vi "FirstOrderFilter.vi"(9 "fps":dbl, 10 "fc":dbl, 11 "Numeric in":dbl) -> (3 "Numeric out":dbl)   [LabVIEW 2017]
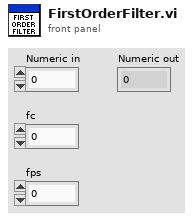
[diagram p1: front panel]
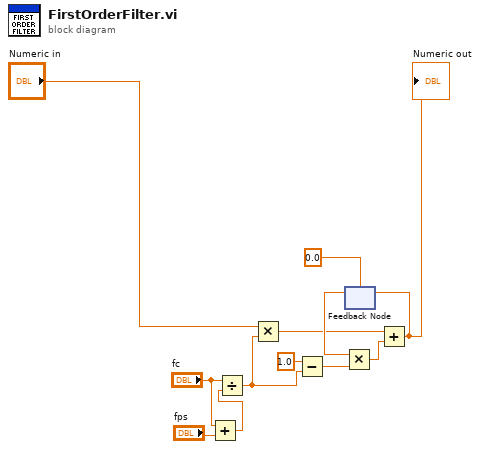
[diagram p0: block diagram]
diagram:
  n1 = Add(x="fc", y="fps") -> (x+y=w9:dbl)
  n2 = Divide(x="fc", y=w9) -> (x/y=w3:dbl)
  n3 = Multiply(x="Numeric in", y=w3) -> (x*y=w6:dbl)
  n4 = Subtract(x=1.0, y=w3) -> (x-y=w4:dbl)
  n5 = feedback #1(0.0) -> (w7:dbl)
  n6 = Multiply(x=w7, y=w4) -> (x*y=w5:dbl)
  n7 = Add(x=w6, y=w5) -> (x+y=w12:dbl)
  "Numeric out" <- w12
  n8 = feedback-in #1(w12) -> ()
